vi "Roller Control.vi"(9 "Jeffery's Stick":T3, 10 "Ian's Buttons":T2, 11 "Ian's Drive":T1) -> (0 "Roller speed":dbl, 1 "Value":T5, 2 "Jeffrey shoot?":bool, 3 "Ian's shoot?":bool, 4 "Jefferys axes":T1, 6 "Jefferys Buttons":T2)   [LabVIEW 2013]
uses:
  <vilib>/Rock Robotics/WPI/Solenoid/WPI_SolenoidValue.ctl
  <vilib>/Rock Robotics/WPI/Joystick/WPI_JoystickButtonState.ctl
  <vilib>/Rock Robotics/WPI/Joystick/WPI_JoystickDevRef.ctl
  <vilib>/Rock Robotics/WPI/Joystick/WPI_JoystickDeviceEnum.ctl
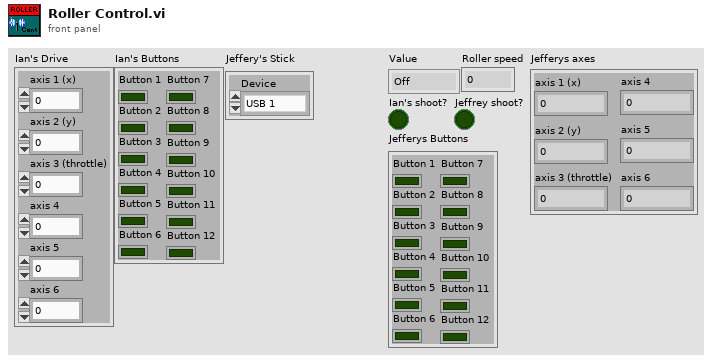
[diagram p1: front panel]
types:
  T1 = cluster{"axis 1 (x)":dbl, "axis 2 (y)":dbl, "axis 3 (throttle)":dbl, "axis 4":dbl, "axis 5":dbl, "axis 6":dbl}
  T2 = typedef "WPI_JoystickButtonState.ctl" = cluster{"Button 1":bool, "Button 2":bool, "Button 3":bool, "Button 4":bool, "Button 5":bool, "Button 6":bool, "Button 7":bool, "Button 8":bool, "Button 9":bool, "Button 10":bool, "Button 11":bool, "Button 12":bool}
  T3 = typedef "WPI_JoystickDevRef.ctl" = cluster{"Device":T4}
  T4 = typedef "WPI_JoystickDeviceEnum.ctl" = enum16{"USB 1", "USB 2", "USB 3", "USB 4", "Kinect 1", "Kinect 2"}
  T5 = typedef "WPI_SolenoidValue.ctl" = enum16{"Off", "On", "Forward", "Reverse"}
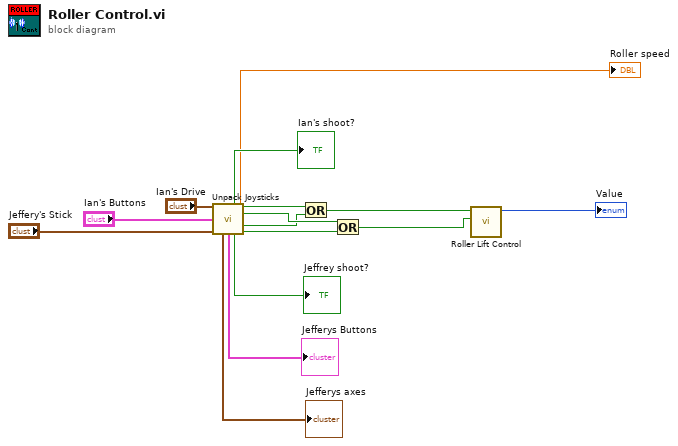
[diagram p0: block diagram]
diagram:
  n1 = call "Unpack Joysticks.vi"("Ian's Drive"="Ian's Drive", "Ian's Buttons"="Ian's Buttons", "Jeffery's Stick"="Jeffery's Stick") -> ("Ian's shoot?"=→"Ian's shoot?":bool, "Ian up"=w12:bool, "Ian down"=w11:bool, "Roller speed(raw)"=→"Roller speed":dbl, "Jeffrey down"=w10:bool, "Jefferys axes"=→"Jefferys axes":T1, "Jefferys Buttons"=→"Jefferys Buttons":T2, "Jeffrey shoot?"=→"Jeffrey shoot?":bool, "Jeffrey up"=w9:bool)  [unwired: 4 in]
  n2 = Or(x=w12, y=w10) -> (x .or. y?=w13:bool)
  n3 = Or(x=w11, y=w9) -> (x .or. y?=w14:bool)
  n4 = call "Roller Lift Control.vi"("Down"=w14, "Up"=w13) -> ("Roller Up/Down"=→"Value":T5)  [unwired: 8 in, 1 out]
